vi "getBounds.vi"(0 "reference":refnum<class "AbstractEdge.lvclass">, 1 "graphics":refnum<class "Graphics.lvclass">, 5 "error in (no error)":errorcluster) -> (14 "reference out":refnum<class "AbstractEdge.lvclass">, 15 "bounds":T1 {"height" format="%.2f"; "width" format="%.2f"; "y" format="%.2f"; "x" format="%.2f"}, 19 "error out":errorcluster)   [LabVIEW 2012, in "AbstractEdge.lvclass"]
doc: "public Rectangle2D getBounds(Graphics2D g2)"
uses:
  <resource>/Framework/Providers/Open_GDS/UML/AbstractEdge_class/AbstractEdge.lvclass
  <resource>/Framework/Providers/Open_GDS/UML/Graphics_class/Graphics.lvclass
  <resource>/Framework/Providers/Open_GDS/UML/General/Rectangle/Rectangle Rectangle2D.ctl
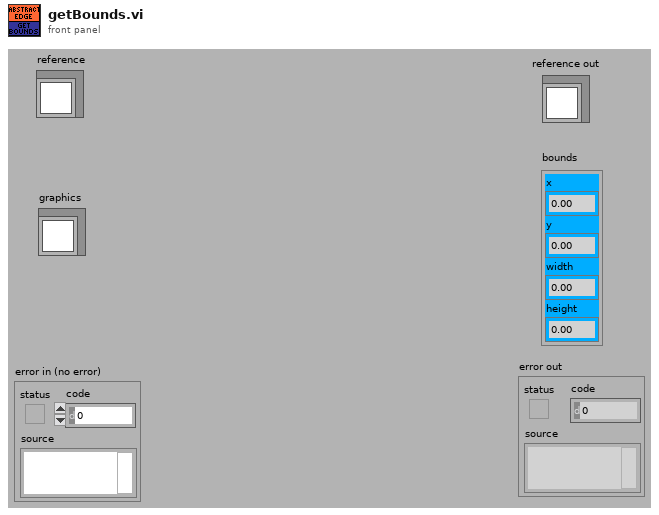
[diagram p1: front panel]
types:
  T1 = typedef "Rectangle Rectangle2D.ctl" = cluster{"x":dbl, "y":dbl, "width":dbl, "height":dbl}
  T2 = typedef "Point Point2D.ctl" = cluster{"x":dbl, "y":dbl}
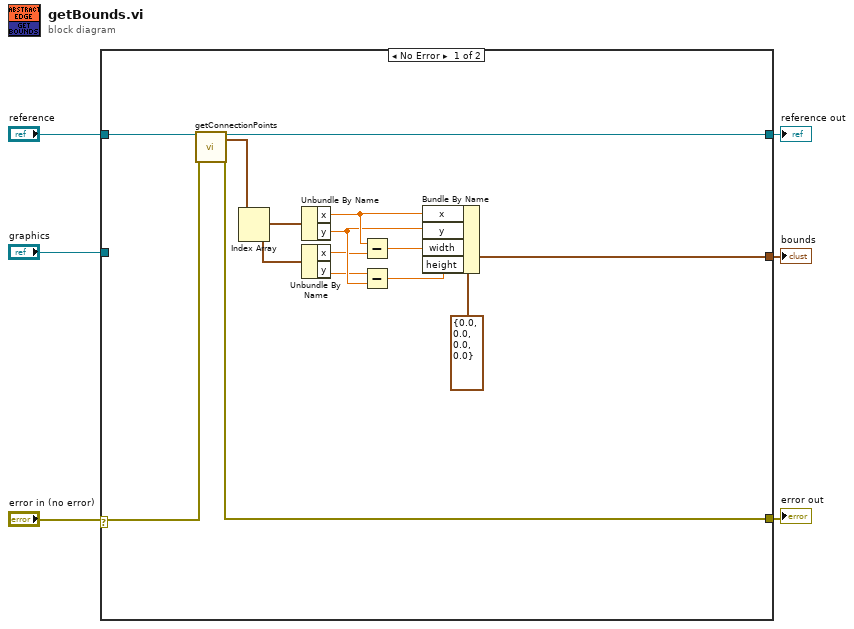
[diagram p0: block diagram]
diagram:
  n1 = case shown="No Error" "error in (no error)" {
    selector: "error in (no error)" -> [w18 w22]
    tunnel: "reference" -> [w21 w23]
    tunnel: [w20 w22] -> w5
    tunnel: [w19 w23] -> w4
    tunnel: "graphics" -> [_ _]
    tunnel: [w17 _] -> w2
    frame No Error {
      n2 = call-dynamic "getConnectionPoints.vi"("reference"=w21, "error in (no error)"=w18) -> ("reference out"=w19:refnum<class "AbstractEdge.lvclass">, "connectionPoints"=w16:T2[], "error out"=w20:errorcluster)  [unwired: 15 in]
      n3 = Index Array(array=w16) -> (element #1=w14:T2, element #2=w13:T2)  [unwired: 2 in]
      n4 = Unbundle By Name(w14) -> ("x"=w12:dbl, "y"=w10:dbl)
      n5 = Unbundle By Name(w13) -> ("x"=w7:dbl, "y"=w9:dbl)
      n6 = Subtract(x=w12, y=w7) -> (x-y=w11:dbl)
      n7 = Subtract(x=w9, y=w10) -> (x-y=w8:dbl)
      n8 = Bundle By Name(cluster=T1 {"x"=0.0, "y"=0.0, "width"=0.0, "height"=0.0} ("bounds"), "x"=w12, "y"=w10, "width"=w11, "height"=w8) -> (w17:T1)
    }
    frame Error {
    }
  }
  "reference out" <- w4
  "error out" <- w5
  "bounds" <- w2
